vi "Client(XML).vi"() -> ()   [LabVIEW 2013, in "OPC UA Demo.lvlib"]
doc: "Demonstrates the use of the <B>OPC UA Client VIs</B> to programmatically create an OPC UA client and connects the OPC UA client to an OPC UA server."
uses:
  OPC UA Demo.lvlib
  <vilib>/OPCUA/NI OPC UA Client.lvlib
  <vilib>/OPCUA/client/Write Int32.vi
  OPCUA XML/OPCUA XML.lvlib
panel:
  in  "Device.Node.Set Point":i32=1000
  out "error out":errorcluster
  out "Waveform Chart":i32(graph)
  in  "stop":bool
  # "Overview: Demonstrates the use of the OPC UA Client VIs to programmatically create an OPC UA client and connects the OPC UA client to an OPC UA server.\nRequirements: \n1. LabVIEW Datalogging and Supervisory Control Module or LabVIEW Real-Time Module\n2. (Real-Time Module) RT target\nInstructions:\nRun the VI."
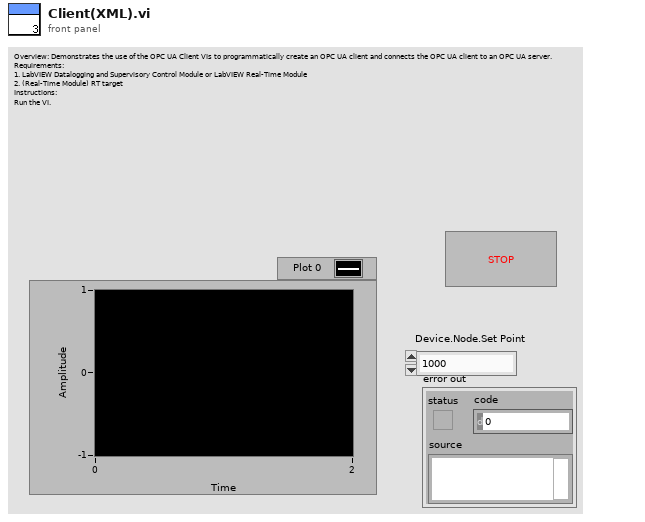
[diagram p1: front panel]
types:
  T1 = cluster{"Item URL":string, "Item Value":variant, "Timestamp":timestamp, "DataType":u32, "status code":u32}[]
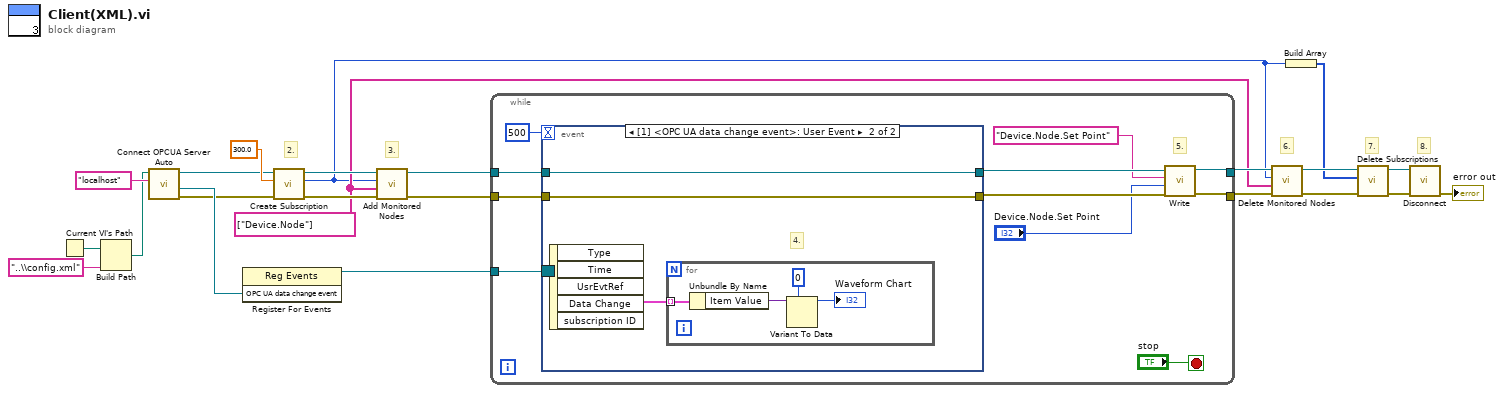
[diagram p0: block diagram]
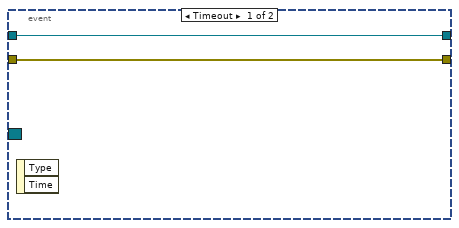
[diagram p2: hidden frame]
diagram:
  w11 = string[] ["Device.Node"] ("array of node path")
  # "7."
  # "8."
  # "6."
  # "3."
  # "2."
  n1 = Current VI's Path() -> (path=w3:path)
  n2 = Build Path(base path=w3, name or relative path="..\\config.xml") -> (appended path=w1:path)
  n3 = call "Connect OPCUA Server Auto.vi"("Server IP"="localhost", "XML config File Path"=w1) -> ("Error Out"=w5:errorcluster, "OPC UA data change event"=w6:refnum<user-event>, "OPC UA client refnum"=w7:refnum<k21>)  [unwired: 5 in, 2 out]
  n4 = register-events(w6) -> (reference out=w21:refnum<event-registration>)  [unwired: 2 in, 1 out]
  n5 = call <vilib>:"Create Subscription.vi"("error in (no error)"=w5, "update rate (1000 ms)"=300.0, "OPC UA client refnum in"=w7) -> ("error out"=w22:errorcluster, "subscription ID out"=w10:u32, "OPC UA client refnum out"=w23:refnum<k21>)  [unwired: 6 in]
  n6 = call <vilib>:"Add Monitored Nodes.vi"("error in (no error)"=w22, "array of node path"=w11, "subscription ID in"=w10, "OPC UA client refnum in"=w23) -> ("error out"=w19:errorcluster, "OPC UA client refnum out"=w20:refnum<k21>)  [unwired: 5 in, 1 out]
  n7 = while {
    tunnel: w21 -> [w34]
    tunnel: w20 -> [w32]
    tunnel: w19 -> [w31]
    tunnel: [w27] -> w17
    tunnel: [w29] -> w18
    stop <- "stop" stop-if-true
    # "5."
    n8 = event shown="[1] <OPC UA data change event>: User Event" {
      selector: w34 -> [_ _]
      dyn-events: _ -> [_ _]
      timeout: 500 -> [_ _]
      tunnel: w32 -> [w36 w39]
      tunnel: w31 -> [w35 w38]
      tunnel: [w36 w39] -> w30
      tunnel: [w35 w38] -> w28
      event Timeout {
        n9 = event-data() -> ()  [unwired: 1 in, 2 out]
      }
      event User Event {
        # "4."
        n10 = event-data() -> ("Data Change"=w37:T1)  [unwired: 1 in, 4 out]
        n11 = for {
          tunnel: w37 -> [w43] mode=indexing
          n12 = Unbundle By Name(w43) -> ("Item Value"=w42:variant)
          n13 = Variant To Data(type=0, Variant=w42) -> (data=→"Waveform Chart":i32)  [unwired: 1 in, 1 out]
        }
      }
    }
    n14 = call-poly <vilib>:"Write.vi"("error in (no error)"=w28, "value"="Device.Node.Set Point", "node path"="Device.Node.Set Point", "OPC UA client refnum in"=w30) -> ("error out"=w27:errorcluster, "OPC UA client refnum out"=w29:refnum<k21>)  [unwired: 5 in, 1 out]
  }
  n15 = call <vilib>:"Delete Monitored Nodes.vi"("error in (no error)"=w17, "array of node path"=w11, "subscription ID in"=w10, "OPC UA client refnum in"=w18) -> ("error out"=w15:errorcluster, "OPC UA client refnum out"=w16:refnum<k21>)  [unwired: 4 in, 2 out]
  n16 = Build Array(w10) -> (w9:u32[])
  n17 = call <vilib>:"Delete Subscriptions.vi"("error in (no error)"=w15, "array of subscription ID"=w9, "OPC UA client refnum in"=w16) -> ("error out"=w13:errorcluster, "OPC UA client refnum out"=w14:refnum<k21>)  [unwired: 6 in, 1 out]
  n18 = call <vilib>:"Disconnect.vi"("error in (no error)"=w13, "OPC UA client refnum in"=w14) -> ("error out"=→"error out":errorcluster)  [unwired: 9 in]
